vi "send_image.vi"(7 "force sending?":bool, 8 "error in (no error)":errorcluster, 9 "image finished?":bool=TRUE, 10 "image (channels)":refnum<class "Image.lvclass">[](array[class]), 11 "GenericToplevelComponent in":refnum<class "GenericToplevelComponent.lvclass">) -> (0 "error out":errorcluster, 3 "GenericToplevelComponent out":refnum<class "GenericToplevelComponent.lvclass">, 4 "# elements in queue":i32)   [LabVIEW 2010, in "GenericToplevelComponent.lvclass"]
uses:
  GenericToplevelComponent.lvclass
  Image/Image/Image.lvclass
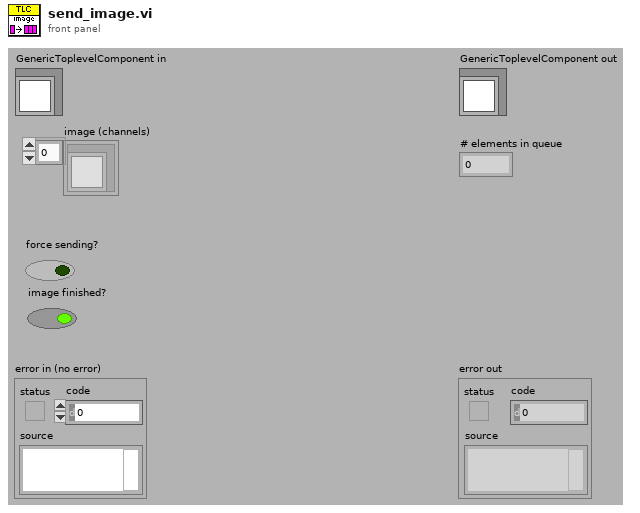
[diagram p1: front panel]
types:
  T1 = typedef "Image Type" = u32
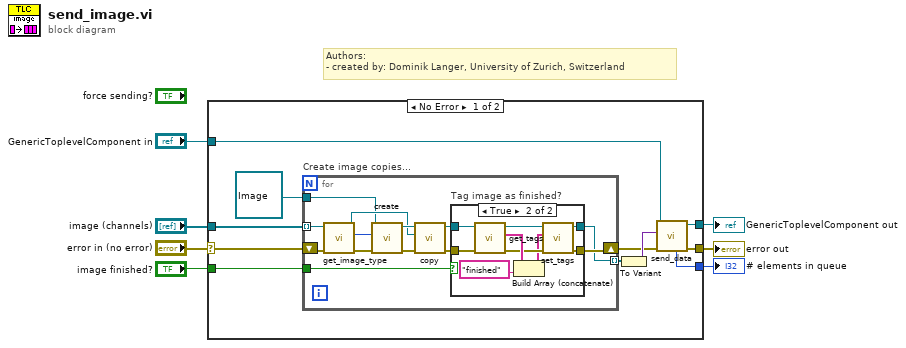
[diagram p0: block diagram]
diagram:
  # "Authors: \n- created by: Dominik Langer, University of Zurich, Switzerland"
  n1 = case shown="No Error" "error in (no error)" {
    selector: "error in (no error)" -> [w18 w44]
    tunnel: [w13 w44] -> w6
    tunnel: [w10 w43] -> w4
    tunnel: "GenericToplevelComponent in" -> [w11 w43]
    tunnel: "image (channels)" -> [w9 _]
    tunnel: "image finished?" -> [w16 _]
    tunnel: [w12 _] -> w1
    frame No Error {
      n2 = for "Create image copies..." {
        tunnel: w9 -> [w27] mode=indexing
        shift-right: [w22] -> w14
        shift-left: w18 -> [w29]
        tunnel: [w20] -> w17 mode=indexing
        tunnel: refnum<class "Image.lvclass"> refnum ("Image.lvclass") -> [w24]
        tunnel: w16 -> [w19]
        n3 = call-dynamic "get_image_type.vi"("error in (no error)"=w29, "Image.lvclass in"=w27) -> ("error out"=w28:errorcluster, "Image Type"=w25:T1, "Image.lvclass out"=w26:refnum<class "Image.lvclass">)  [unwired: 7 out]
        n4 = call "create.vi"("error in (no error)"=w28, "Image Type"=w25, "Image in"=w24) -> ("error out"=w31:errorcluster, "Image out"=w30:refnum<class "Image.lvclass">)  [unwired: 1 in, 6 out]
        n5 = call "copy.vi"("error in (no error)"=w31, "image to copy (source)"=w26, "Image in (target)"=w30) -> ("error out"=w23:errorcluster, "Image out"=w21:refnum<class "Image.lvclass">)  [unwired: 7 out]
        n6 = case "Tag image as finished?" shown="True" w19 {
          tunnel: w23 -> [w33 w40]
          tunnel: [w33 w39] -> w22
          tunnel: w21 -> [w32 w37]
          tunnel: [w32 w36] -> w20
          frame False {
          }
          frame True {
            n7 = call "get_tags.vi"("error in (no error)"=w40, "Image.lvclass in"=w37) -> ("error out"=w41:errorcluster, "tags"=w42:string[], "Image.lvclass out"=w38:refnum<class "Image.lvclass">)  [unwired: 7 in]
            n8 = Build Array (concatenate)(w42, "finished" ("String")) -> (w35:string[])
            n9 = call "set_tags.vi"("error in (no error)"=w41, "tags"=w35, "Image.lvclass in"=w38) -> ("error out"=w39:errorcluster, "Image.lvclass out"=w36:refnum<class "Image.lvclass">)  [unwired: 7 in]
          }
        }
      }
      n10 = To Variant(anything=w17) -> (Variant=w15:variant)
      n11 = call-dynamic "send_data.vi"("error in (no error)"=w14, "data"=w15, "GenericToplevelComponent in"=w11) -> ("error out"=w13:errorcluster, "GenericToplevelComponent out"=w10:refnum<class "GenericToplevelComponent.lvclass">, "# elements in queue"=w12:i32)  [unwired: 6 in]
    }
    frame Error {
    }
  }
  "error out" <- w6
  "GenericToplevelComponent out" <- w4
  "# elements in queue" <- w1
